vi "RANGE Get COM Ports.vi"(0 "all rows":string[][](array[string]), 1 "Meter 1 Present":bool, 2 "Meter 2 Present":bool, 3 "Meter 3 Present":bool, 4 "Meter 4 Present":bool, 5 "Error In":errorcluster, 6 "Meter 5 Present":bool, 8 "Meter 6 Present":bool) -> (12 "Meter 1":refnum<visa-resource-name>, 14 "Meter 2":refnum<visa-resource-name>, 15 "Meter 3":refnum<visa-resource-name>, 16 "Meter 4":refnum<visa-resource-name>, 17 "Meter 5":refnum<visa-resource-name>, 18 "Meter 6":refnum<visa-resource-name>, 19 "Error Out":errorcluster)   [LabVIEW 2018]
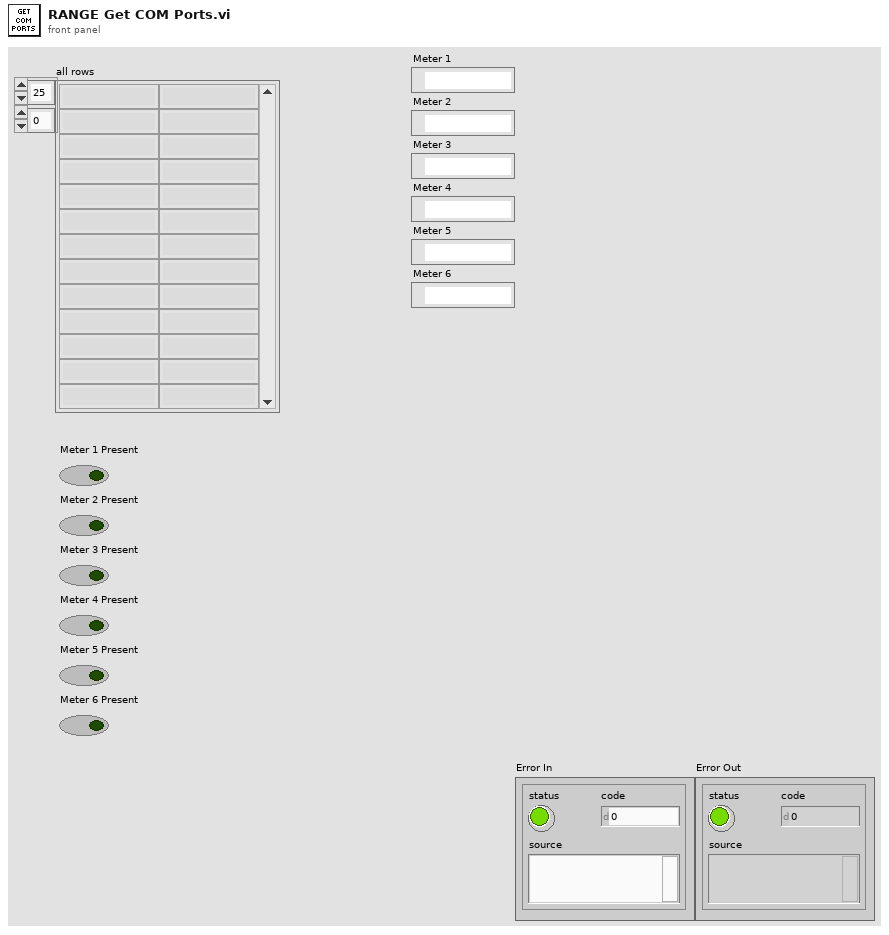
[diagram p1: front panel]
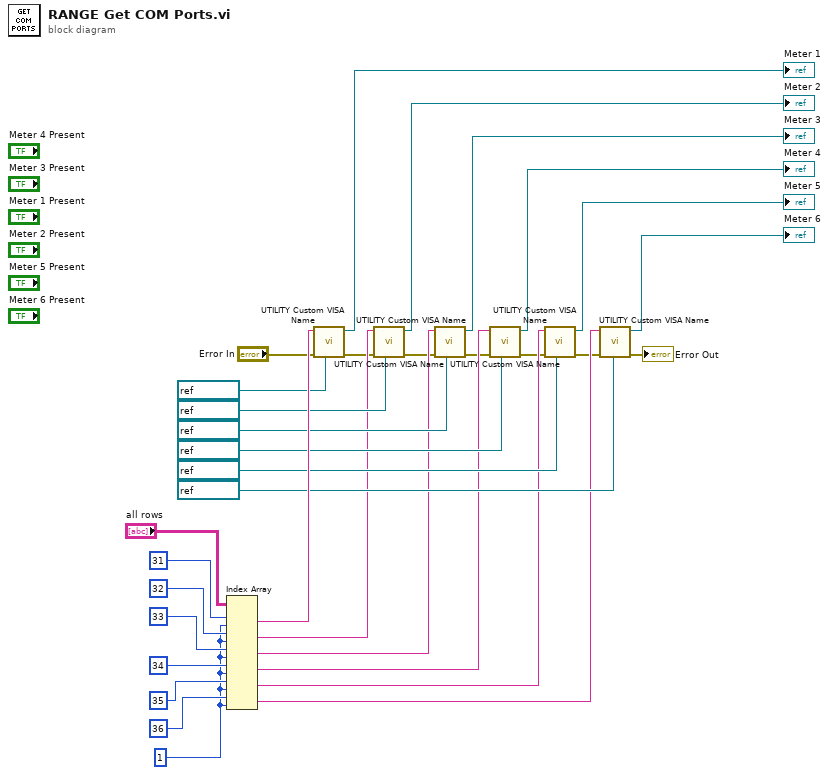
[diagram p0: block diagram]
diagram:
  w28 = 1 ("disabled index (col)")
  n1 = Index Array(array="all rows", index (row) #1=31 ("disabled index (row)"), index (col) #1=w28, index (row) #2=32 ("disabled index (row)"), index (col) #2=w28, index (row) #3=33 ("disabled index (row)"), index (col) #3=w28, index (row) #4=34 ("disabled index (row)"), index (col) #4=w28, index (row) #5=35 ("disabled index (row)"), index (col) #5=w28, index (row) #6=36 ("disabled index (row)"), index (col) #6=w28) -> (element #1=w25:string, element #2=w12:string, element #3=w11:string, element #4=w10:string, element #5=w9:string, element #6=w8:string)
  n2 = call "UTILITY Custom VISA Name.vi"("Default VISA Name"=refnum<visa-resource-name> "COM3", "Error In"="Error In", "Input Name (String)"=w25) -> ("Error Out"=w7:errorcluster, "Name (VISA)"=→"Meter 1":refnum<visa-resource-name>)  [unwired: 7 in]
  n3 = call "UTILITY Custom VISA Name.vi"("Default VISA Name"=refnum<visa-resource-name> "COM4" ("Meter 1.Meter Visa"), "Error In"=w7, "Input Name (String)"=w12) -> ("Error Out"=w6:errorcluster, "Name (VISA)"=→"Meter 2":refnum<visa-resource-name>)  [unwired: 7 in]
  n4 = call "UTILITY Custom VISA Name.vi"("Default VISA Name"=refnum<visa-resource-name> "COM5" ("Meter 1.Meter Visa"), "Error In"=w6, "Input Name (String)"=w11) -> ("Error Out"=w5:errorcluster, "Name (VISA)"=→"Meter 3":refnum<visa-resource-name>)  [unwired: 7 in]
  n5 = call "UTILITY Custom VISA Name.vi"("Default VISA Name"=refnum<visa-resource-name> "COM6" ("Meter 1.Meter Visa"), "Error In"=w5, "Input Name (String)"=w10) -> ("Error Out"=w4:errorcluster, "Name (VISA)"=→"Meter 4":refnum<visa-resource-name>)  [unwired: 7 in]
  n6 = call "UTILITY Custom VISA Name.vi"("Default VISA Name"=refnum<visa-resource-name> "COM7" ("Meter 1.Meter Visa"), "Error In"=w4, "Input Name (String)"=w9) -> ("Error Out"=w3:errorcluster, "Name (VISA)"=→"Meter 5":refnum<visa-resource-name>)  [unwired: 7 in]
  n7 = call "UTILITY Custom VISA Name.vi"("Default VISA Name"=refnum<visa-resource-name> "COM8" ("Meter 1.Meter Visa"), "Error In"=w3, "Input Name (String)"=w8) -> ("Error Out"=→"Error Out":errorcluster, "Name (VISA)"=→"Meter 6":refnum<visa-resource-name>)  [unwired: 7 in]
